vi "GetDLLPath.vi"(9 "DllName_32bit":string, 10 "PathToDLL":path, 11 "DllName_64bit":string) -> (2 "file exists?":bool, 3 "DLLPath":path)   [LabVIEW 2017]
uses:
  <vilib>/Utility/sysdir.llb/System Directory Type.ctl
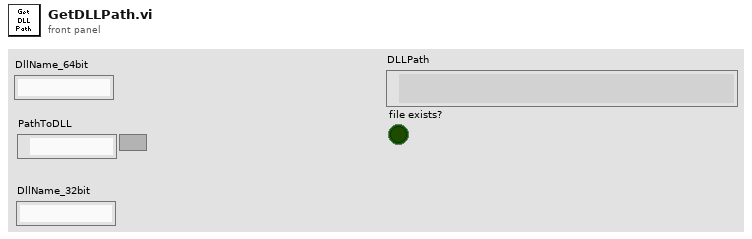
[diagram p1: front panel]
types:
  T1 = typedef "System Directory Type.ctl" = i32
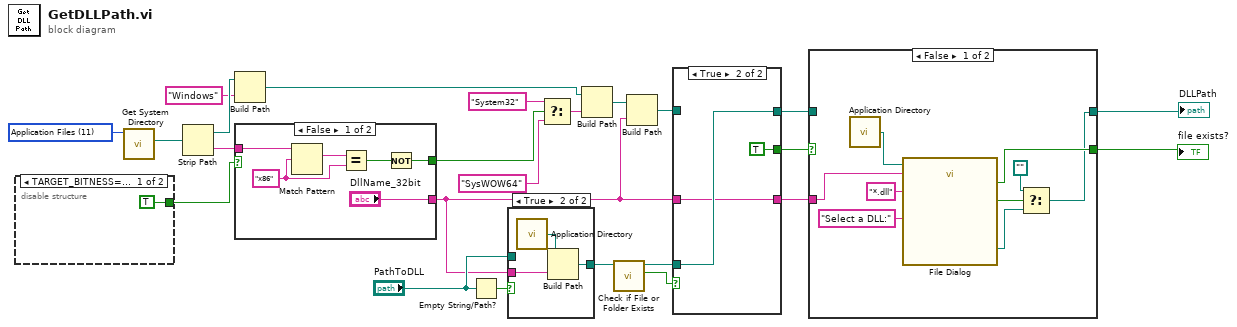
[diagram p0: block diagram]
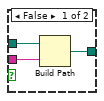
[diagram p3: hidden frame]
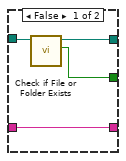
[diagram p4: hidden frame]
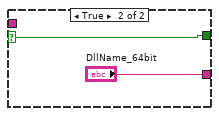
[diagram p5: hidden frame]
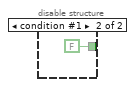
[diagram p6: hidden frame]
diagram:
  w24 = T1 11 items=["User Home"=0, "User Desktop"=1, "User Documents"=2, "User Application Data"=3, "User Preferences"=4, "User Temporary"=5, "Public Documents"=6, "Public Application Data"=7, "Public Preferences"=8, "Public Cache"=13, "System Core Libraries"=9, "System Installed Libraries"=10, "Application Files"=11, "Boot Volume Root"=12] ("system directory type")
  n1 = disable-structure shown="TARGET_BITNESS==64, Default" {
    disable-tunnel: [TRUE FALSE] -> w16
    frame condition #0 (active) {
    }
    frame condition #1 {
    }
  }
  n2 = call <vilib>:"Get System Directory.vi"("system directory type"=w24) -> ("system directory"=w23:path)  [unwired: 10 in]
  n3 = Strip Path(path=w23) -> (stripped path=w22:path, name=w14:string)
  n4 = Build Path(base path=w22, name or relative path="Windows") -> (appended path=w20:path)
  n5 = case shown="False" w16 {
    selector: w16 -> [_ w34]
    tunnel: [w28 w34] -> w15
    tunnel: w14 -> [w32 _]
    tunnel: ["DllName_32bit" "DllName_64bit"] -> w1
    frame False {
      w31 = "x86" ("regular expression")
      n6 = Match Pattern(string=w32, regular expression=w31) -> (match substring=w30:string)  [unwired: 1 in, 3 out]
      n7 = Equal?(x=w30, y=w31) -> (x = y?=w29:bool)
      n8 = Not(x=w29) -> (.not. x?=w28:bool)
    }
    frame True {
    }
  }
  n9 = Empty String/Path?(string/path="PathToDLL") -> (empty?=w9:bool)
  n10 = case shown="True" w9 {
    tunnel: "PathToDLL" -> [w37 _]
    tunnel: w1 -> [w36 w39]
    tunnel: [w35 w38] -> w7
    frame False {
      n11 = Build Path(base path=w37, name or relative path=w36) -> (appended path=w35:path)
    }
    frame True {
      n12 = call <vilib>:"Application Directory.vi"() -> ("Application Directory"=w40:path)
      n13 = Build Path(base path=w40, name or relative path=w39) -> (appended path=w38:path)
    }
  }
  n14 = Select(t="System32" ("name or relative path"), s=w15, f="SysWOW64" ("name or relative path")) -> (s? t:f=w18:string)
  n15 = Build Path(base path=w20, name or relative path=w18) -> (appended path=w13:path)
  n16 = call <vilib>:"Check if File or Folder Exists.vi"("path"=w7) -> ("file or folder exists?"=w12:bool, "dup path"=w10:path)  [unwired: 8 in, 1 out]
  n17 = Build Path(base path=w13, name or relative path=w1) -> (appended path=w11:path)
  n18 = case shown="True" w12 {
    tunnel: w11 -> [w44 _]
    tunnel: [w43 TRUE ("file or folder exists?")] -> w6
    tunnel: [w42 w47] -> w5
    tunnel: w10 -> [_ w47]
    tunnel: [w41 w45] -> w2
    tunnel: w1 -> [w41 w45]
    frame False {
      n19 = call <vilib>:"Check if File or Folder Exists.vi"("path"=w44) -> ("file or folder exists?"=w43:bool, "dup path"=w42:path)  [unwired: 8 in, 1 out]
    }
    frame True {
    }
  }
  n20 = case shown="False" w6 {
    selector: w6 -> [_ w57]
    tunnel: w5 -> [_ w58]
    tunnel: [w49 w58] -> w4
    tunnel: [w52 w57] -> w3
    tunnel: w2 -> [w55 _]
    frame False {
      n21 = call <vilib>:"Application Directory.vi"() -> ("Application Directory"=w56:path)
      n22 = call "File Dialog"("start path"=w56, "prompt"="Select a DLL:", "default name"=w55, "pattern (all files)"="*.dll") -> ("selected path"=w50:path, "exists"=w52:bool, "cancelled"=w51:bool)  [unwired: 8 in, 1 out]
      n23 = Select(t=path "", s=w51, f=w50) -> (s? t:f=w49:path)
    }
    frame True {
    }
  }
  "DLLPath" <- w4
  "file exists?" <- w3
